vi "oa_Extract First Cycle Data (N Channels).vi"(0 "resampled signal":cluster{"r0":dbl, "dr":dbl, "Y":dbl[]}[](array[cluster]) {"r0" format="%.2p"; "dr" format="%.2p"; "Y" format="%.2f"}, 1 "reset? (True)":bool=TRUE, 5 "speed profile":T1 {"speed [RPM]" format="%.2f"; "time [s]" format="%.2f"}, 7 "interpolated pulse positions":dbl[](array[numeric]) format="%.2f", 11 "error in (no error)":errorcluster) -> (4 "resampled signal out":cluster{"r0":dbl, "dr":dbl, "Y":dbl[]}[](array[cluster]) {"r0" format="%.2p"; "dr" format="%.2p"; "Y" format="%.2f"}, 6 "waveform reference data":cluster{"r0":dbl, "dr":dbl, "Y":dbl[]}[](array[cluster]) {"r0" format="%.2p"; "dr" format="%.2p"; "Y" format="%.2f"}, 15 "error out":errorcluster)   [LabVIEW 2017, in "SoundVib_RefDataProcess.lvlib"]
uses:
  <vilib>/addons/Sound and Vibration/Order Analysis/Referece Data Processing/SoundVib_RefDataProcess.lvlib
  <vilib>/addons/Sound and Vibration/Order Analysis/Tach Process/SubVIs/speed profile.ctl
  <vilib>/addons/Sound and Vibration/Order Analysis/Resample Order Tracking/SoundVib_Resampling.lvlib
  <vilib>/addons/Sound and Vibration/Order Analysis/Tach Process/SoundVib_TachProcess.lvlib
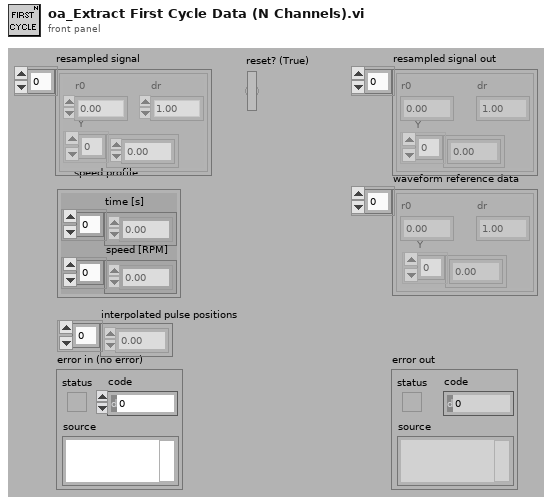
[diagram p1: front panel]
types:
  T1 = typedef "SoundVib_TachProcess.lvlib/speed profile.ctl" = cluster{"time [s]":dbl[], "speed [RPM]":dbl[]}
  T2 = enum16{"averaged samples", "initial samples", "final samples"}
  T3 = cluster{"r0":dbl, "dr":dbl, "reference data":dbl[]}[]
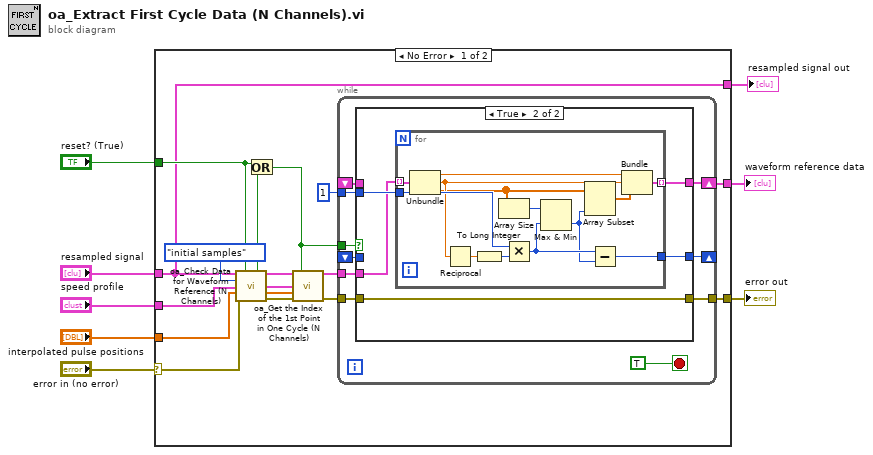
[diagram p0: block diagram]
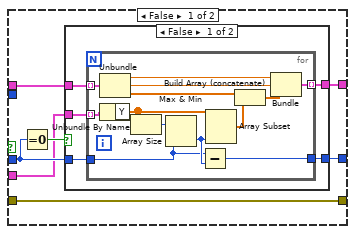
[diagram p2: hidden frame]
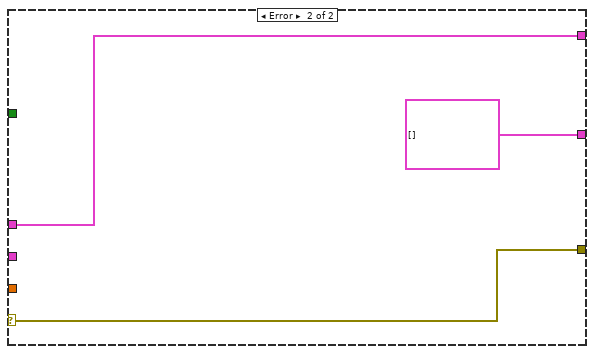
[diagram p4: hidden frame]
diagram:
  n1 = case shown="No Error" "error in (no error)" {
    selector: "error in (no error)" -> [w13 w83]
    tunnel: [w25 T3 []] -> w8
    tunnel: [w24 w83] -> w7
    tunnel: "speed profile" -> [w17 _]
    tunnel: "reset? (True)" -> [w16 _]
    tunnel: "resampled signal" -> [w9 w81]
    tunnel: "interpolated pulse positions" -> [w10 _]
    tunnel: [w9 w81] -> w1
    frame No Error {
      n2 = call <vilib>:"oa_Check Data for Waveform Reference (N Channels).vi"("resampled signal"=w9, "reset? (True)"=w16, "select reference data"=T2."initial samples", "speed profile"=w17, "interpolated pulse positions"=w10, "error in (no error)"=w13) -> ("reset"=w22:bool, "resampled data out"=w19:cluster{"r0":dbl, "dr":dbl, "Y":dbl[]}[], "speed profile out"=w21:T1, "interpolated pulse positions out"=w20:dbl[], "error out"=w18:errorcluster)  [unwired: 2 in, 3 out]
      n3 = Or(x=w16, y=w22) -> (x .or. y?=w23:bool)
      n4 = call <vilib>:"oa_Get the Index of the 1st Point in One Cycle (N Channels).vi"("resampled signal"=w19, "reset? (True)"=w23, "speed profile"=w21, "interpolated pulse positions"=w20, "error in (no error)"=w18) -> ("resampled signal out"=w14:cluster{"r0":dbl, "dr":dbl, "Y":dbl[]}[], "error out"=w15:errorcluster)  [unwired: 8 in, 1 out]
      n5 = while {
        tunnel: w23 -> [w28]
        tunnel: 1 -> [w34]
        shift-right: [w33] -> w25
        shift-left: _ -> [w31]
        shift-right: [w32] -> _
        shift-left: _ -> [w30]
        tunnel: [w29] -> w24
        tunnel: w15 -> [w27]
        tunnel: w14 -> [w26]
        stop <- TRUE stop-if-true
        n6 = case shown="True" w28 {
          tunnel: w27 -> [w37 w63]
          tunnel: w34 -> [_ w67]
          tunnel: [w38 w66] -> w33
          tunnel: [w42 w65] -> w32
          tunnel: w31 -> [w41 _]
          tunnel: w30 -> [w40 _]
          tunnel: [w37 w63] -> w29
          tunnel: w26 -> [w36 w64]
          frame False {
            n7 = Equal To 0?(x=w40) -> (x = 0?=w39:bool)
            n8 = case shown="False" w39 {
              tunnel: [w47 w61] -> w42
              tunnel: w41 -> [w46 w62]
              tunnel: w40 -> [w45 w61]
              tunnel: [w44 w62] -> w38
              tunnel: w36 -> [w43 _]
              frame False {
                n9 = for {
                  tunnel: [w59] -> w47
                  tunnel: w46 -> [w57] mode=indexing
                  tunnel: w45 -> [w56]
                  tunnel: [w51] -> w44 mode=indexing
                  tunnel: w43 -> [w50] mode=indexing
                  n10 = Unbundle(w57) -> ("r0"=w52:dbl, "dr"=w53:dbl, w49:dbl[])
                  n11 = Unbundle By Name(w50) -> ("Y"=w48:dbl[])
                  n12 = Array Size(array=w48) -> (size(s)=w60:i32)
                  n13 = Max & Min(x=w60, y=w56) -> (min(x,y)=w58:i32)  [unwired: 1 out]
                  n14 = Subtract(x=w56, y=w58) -> (x-y=w59:i32)
                  n15 = Array Subset(array=w48, length=w58) -> (w55:dbl[])  [unwired: 1 in]
                  n16 = Build Array (concatenate)(w49, w55) -> (w54:dbl[])
                  n17 = Bundle("r0"=w52, "dr"=w53, w54) -> (w51:cluster{"r0":dbl, "dr":dbl, dbl[]})  [unwired: 1 in]
                }
              }
              frame True {
              }
            }
          }
          frame True {
            n18 = for {
              tunnel: w67 -> [w80]
              tunnel: [w73] -> w66 mode=indexing
              tunnel: [w72] -> w65
              tunnel: w64 -> [w71] mode=indexing
              n19 = Unbundle(w71) -> ("r0"=w70:dbl, "dr"=w69:dbl, "Y"=w68:dbl[])
              n20 = Reciprocal(x=w69) -> (1/x=w79:dbl)
              n21 = To Long Integer(number=w79) -> (32bit integer=w78:i32)
              n22 = Array Size(array=w68) -> (size(s)=w77:i32)
              n23 = Multiply(x=w80, y=w78) -> (x*y=w76:i32)
              n24 = Max & Min(x=w77, y=w76) -> (min(x,y)=w75:i32)  [unwired: 1 out]
              n25 = Array Subset(array=w68, length=w75) -> (w74:dbl[])  [unwired: 1 in]
              n26 = Subtract(x=w76, y=w75) -> (x-y=w72:i32)
              n27 = Bundle("r0"=w70, "dr"=w69, w74) -> (w73:cluster{"r0":dbl, "dr":dbl, dbl[]})  [unwired: 1 in]
            }
          }
        }
      }
    }
    frame Error {
    }
  }
  "error out" <- w7
  "waveform reference data" <- w8
  "resampled signal out" <- w1
